vi "Init.vi"(8 "error in (no error)":errorcluster) -> (0 "error out":errorcluster, 3 "controller out":refnum<class "Temperature Controller.lvclass">)   [LabVIEW 2019, in "Temperature Controller.lvclass"]
uses:
  Temperature Controller.lvclass
  Temperature Controller.lvclass/Temperature Controller.ctl
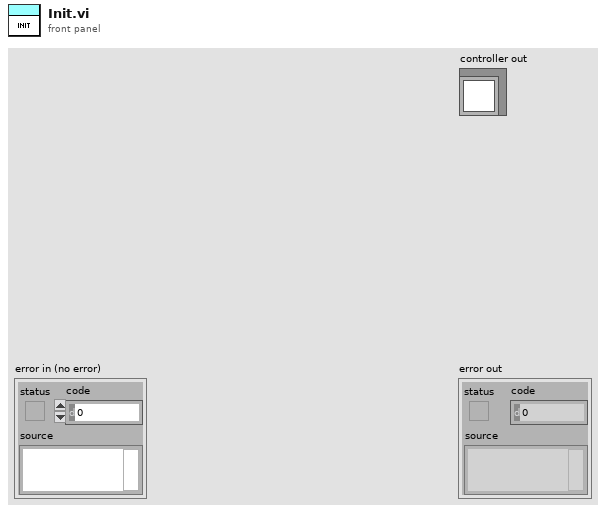
[diagram p1: front panel]
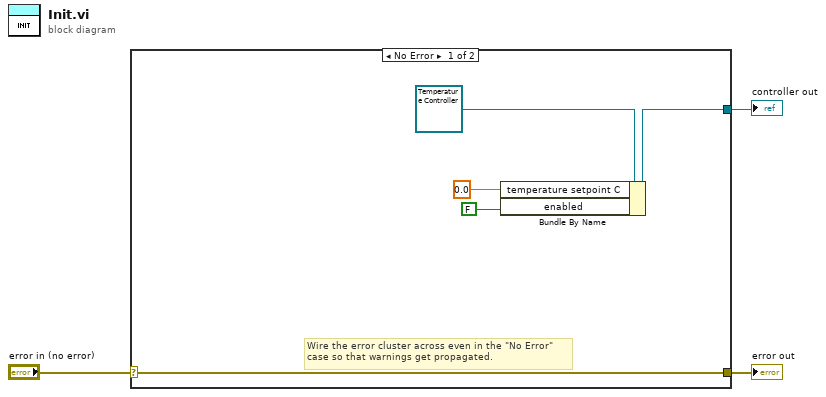
[diagram p0: block diagram]
diagram:
  n1 = case shown="No Error" "error in (no error)" {
    selector: "error in (no error)" -> [w8 w9]
    tunnel: [w8 w9] -> w2
    tunnel: [w6 _] -> w1
    frame No Error {
      # "Wire the error cluster across even in the \"No Error\"\ncase so that warnings get propagated."
      n2 = Bundle By Name(cluster=refnum<class "Temperature Controller.lvclass"> refnum ("TemperatureSensor out"), "temperature setpoint C"=0.0 ("temperature setpoint"), "enabled"=FALSE) -> (w6:refnum<class "Temperature Controller.lvclass">)
    }
    frame Error {
    }
  }
  "error out" <- w2
  "controller out" <- w1
